vi "DisplayStriptestData.vi"(5 "min scale array":i32[](array[numeric]), 6 "max scale array":i32[](array[numeric]), 7 "# probed":i32, 8 "Display Stats?":bool, 9 "Thresholds":T2, 10 "Region":i32) -> (0 "Defects":i32[][](graph), 1 "Resistance [MW]":cluster{u32, i32, "Array OUT":dbl[]}(graph), 2 "Capacitance [pF]":cluster{u32, i32, "Array OUT":dbl[]}(graph), 3 "Current [nA]":cluster{u32, i32, "Array OUT":dbl[]}(graph), 4 "Strip Quality Data":T1 {"pass Rate in %" format="%.2f"})   [LabVIEW 2019]
panel:
  out "max scale":i32
  out "min scale":i32
  # "Current [nA]:"
  # "Capacitance [pF]:"
  # "Resistance [MW]:"
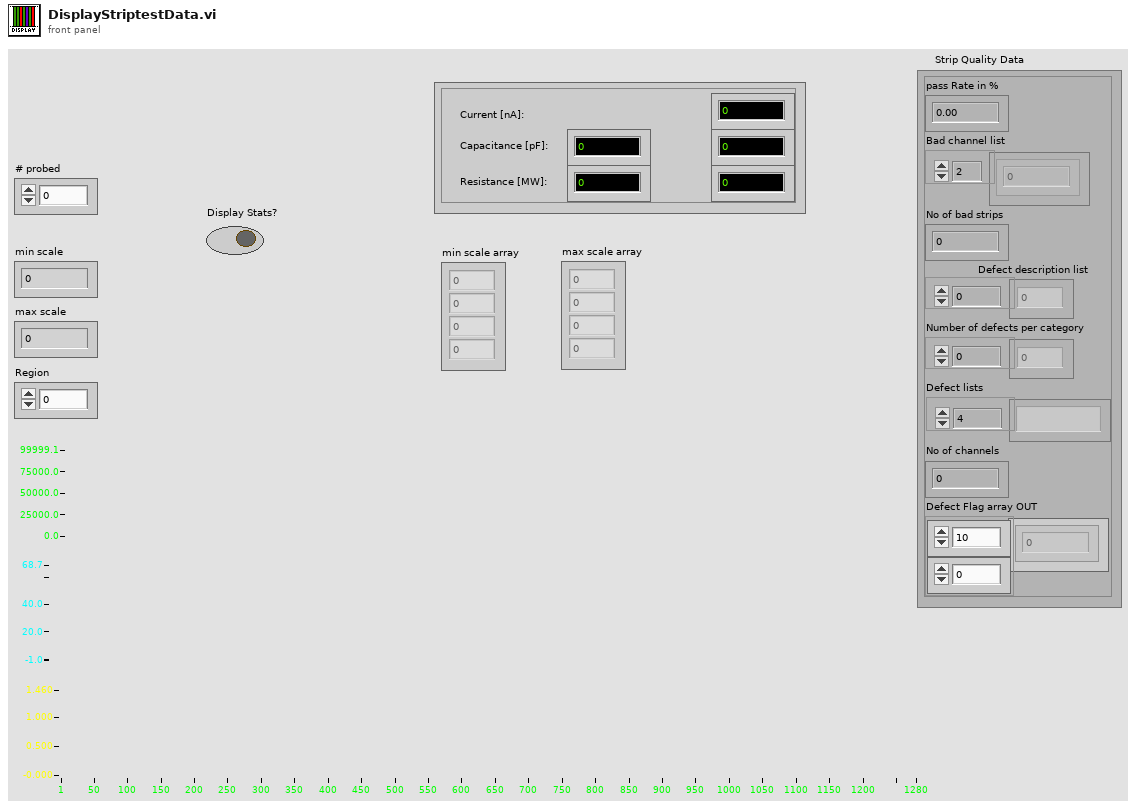
[diagram p1: front panel]
types:
  T1 = cluster{"pass Rate in %":dbl, "Bad channel list":i32[], "No of bad strips":i32, "Defect description list":i32[], "Number of defects per category":i32[], "Defect lists":string[], "No of channels":i32, "Defect Flag array OUT":i32[][]}
  T2 = cluster{"Current [nA]":dbl, "Cap_Lo":dbl, "Cap_Hi":dbl, "Res_Hi":dbl, "Res_Lo":dbl}
  T3 = enum16{"Reset", "Read Array", "Read Element", "Write Element", "Write Array", "Add Element", "Add Array"}
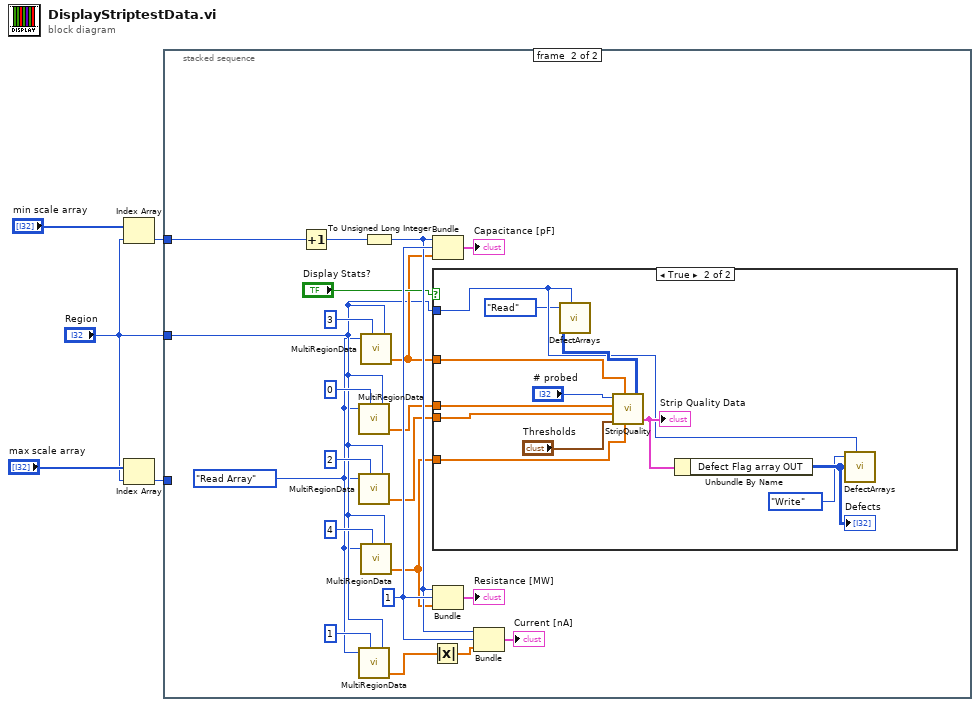
[diagram p0: block diagram]
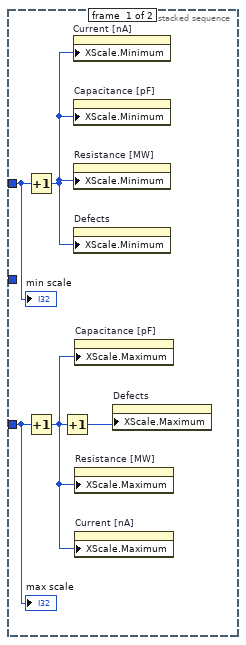
[diagram p2: hidden frame]
diagram:
  n1 = Index Array(array="min scale array", index="Region") -> (element=w4:i32)
  n2 = Index Array(array="max scale array", index="Region") -> (element=w2:i32)
  n3 = stacked-sequence {
    tunnel: w4 -> [w10 w13]
    tunnel: w2 -> [w8 _]
    tunnel: "Region" -> [_ w14]
    frame #0 {
      n4 = Increment(x=w10) -> (x+1=w9:i32)
      n5 = Increment(x=w8) -> (x+1=w7:i32)
      n6 = Increment(x=w7) -> (x+1=w6:i32)
      n7 = property on="Current [nA]" class="WFGraph (strict)"("XScale.Minimum"=w9) -> ()  [unwired: 2 in, 2 out]
      n8 = property on="Capacitance [pF]" class="WFGraph (strict)"("XScale.Minimum"=w9) -> ()  [unwired: 2 in, 2 out]
      n9 = property on="Resistance [MW]" class="WFGraph (strict)"("XScale.Minimum"=w9) -> ()  [unwired: 2 in, 2 out]
      n10 = property on="Defects" class="IntGraph (strict)"("XScale.Minimum"=w9) -> ()  [unwired: 2 in, 2 out]
      n11 = property on="Capacitance [pF]" class="WFGraph (strict)"("XScale.Maximum"=w7) -> ()  [unwired: 2 in, 2 out]
      n12 = property on="Resistance [MW]" class="WFGraph (strict)"("XScale.Maximum"=w7) -> ()  [unwired: 2 in, 2 out]
      n13 = property on="Current [nA]" class="WFGraph (strict)"("XScale.Maximum"=w7) -> ()  [unwired: 2 in, 2 out]
      n14 = property on="Defects" class="IntGraph (strict)"("XScale.Maximum"=w6) -> ()  [unwired: 2 in, 2 out]
      "min scale" <- w10
      "max scale" <- w8
    }
    frame #1 {
      w11 = T3."Read Array" ("Action")
      w26 = 1
      n15 = Increment(x=w13) -> (x+1=w12:i32)
      n16 = call "MultiRegionData.vi"("Action"=w11, "Array No."=0, "Region index"=w14) -> ("Array OUT"=w18:dbl[])  [unwired: 3 in, 1 out]
      n17 = call "MultiRegionData.vi"("Action"=w11, "Array No."=2, "Region index"=w14) -> ("Array OUT"=w15:dbl[])  [unwired: 3 in, 1 out]
      n18 = call "MultiRegionData.vi"("Action"=w11, "Array No."=1, "Region index"=w14) -> ("Array OUT"=w21:dbl[])  [unwired: 3 in, 1 out]
      n19 = call "MultiRegionData.vi"("Action"=w11, "Array No."=3, "Region index"=w14) -> ("Array OUT"=w17:dbl[])  [unwired: 3 in, 1 out]
      n20 = call "MultiRegionData.vi"("Action"=w11, "Array No."=4, "Region index"=w14) -> ("Array OUT"=w16:dbl[])  [unwired: 3 in, 1 out]
      n21 = To Unsigned Long Integer(number=w12) -> (unsigned 32bit integer=w25:u32)
      n22 = Absolute Value(x=w21) -> (abs(x)=w20:dbl[])
      n23 = Bundle(w25, w26, "Array OUT"=w17) -> (→"Capacitance [pF]":cluster{u32, i32, "Array OUT":dbl[]})  [unwired: 1 in]
      n24 = case shown="True" "Display Stats?" {
        tunnel: w18 -> [_ w39]
        tunnel: w17 -> [_ w40]
        tunnel: w16 -> [_ w38]
        tunnel: w15 -> [_ w37]
        tunnel: w14 -> [_ w34]
        frame False {
        }
        frame True {
          n25 = call "DefectArrays.vi"("action"=enum16{"Nothing", "Write", "Read", "Initialise"}."Read", "Region Index"=w34) -> ("Defect array OUT"=w41:i32[][])  [unwired: 1 in, 7 out]
          n26 = call "StripQuality.vi"("No of entries"="# probed", "Capacitance Data Array"=w40, "Channel No. Array"=w39, "Pinhole flag array in"=w37, "Resistance data array"=w38, "Thresholds"="Thresholds", "Defect Flag array IN"=w41) -> ("Strip Quality Data"=w36:T1)  [unwired: 1 out]
          "Strip Quality Data" <- w36
          n27 = Unbundle By Name(w36) -> ("Defect Flag array OUT"=w35:i32[][])
          "Defects" <- w35
          n28 = call "DefectArrays.vi"("action"=enum16{"Nothing", "Write", "Read", "Initialise"}."Write", "Region Index"=w34, "Defect array IN"=w35) -> ()  [unwired: 8 out]
        }
      }
      n29 = Bundle(w25, w26, "Array OUT"=w16) -> (→"Resistance [MW]":cluster{u32, i32, "Array OUT":dbl[]})  [unwired: 1 in]
      n30 = Bundle(w25, w26, w20) -> (→"Current [nA]":cluster{u32, i32, dbl[]})  [unwired: 1 in]
    }
  }
